vi "UTIL_SetDigitalStatus.vi"(9 "index":i32, 10 "Digital Status":T1, 11 "Cluster in":refnum<vi>) -> ()   [LabVIEW 2024]
uses:
  Control Definitions/Def_DigitalStatus.ctl
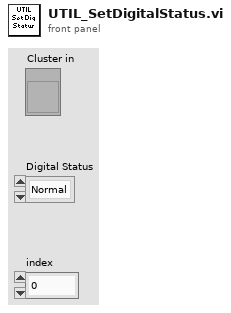
[diagram p1: front panel]
types:
  T1 = typedef "Def_DigitalStatus.ctl" = enum16{"Normal", "Good", "Bad", "Error"}
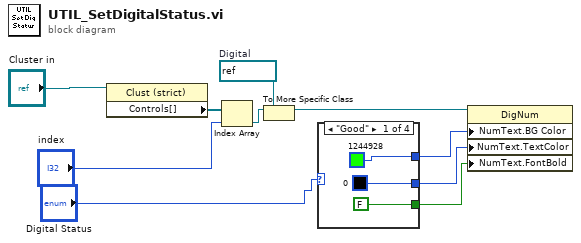
[diagram p0: block diagram]
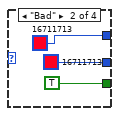
[diagram p2: hidden frame]
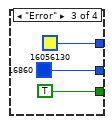
[diagram p3: hidden frame]
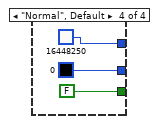
[diagram p4: hidden frame]
diagram:
  w5 = refnum<vi> refnum  # Digital
  n1 = property class="Clust (strict)"(reference="Cluster in") -> ("Controls[]"=w3:refnum<vi>[])  [unwired: 1 in, 2 out]
  n2 = Index Array(array=w3, index="index") -> (element=w4:refnum<vi>)
  n3 = To More Specific Class(target class=w5, reference=w4) -> (specific class reference=w6:refnum<vi>)  [unwired: 1 in, 1 out]
  n4 = case shown="\"Good\"" "Digital Status" {
    tunnel: [u32 0 ("Numeric Text.Colors:FG Color") u32 16711713 ("Numeric Text.Colors:FG Color") u32 16860 ("Numeric Text.Colors:FG Color") u32 0 ("Numeric Text.Colors:FG Color")] -> w9
    tunnel: [FALSE ("Numeric Text.Font:Bold") TRUE ("Numeric Text.Font:Bold") TRUE ("Numeric Text.Font:Bold") FALSE ("Numeric Text.Font:Bold")] -> w10
    tunnel: [u32 1244928 ("Numeric Text.Colors:FG Color") u32 16711713 ("Numeric Text.Colors:FG Color") u32 16056130 ("Numeric Text.Colors:FG Color") u32 16448250 ("Numeric Text.Colors:FG Color")] -> w8
    frame "Good" {
    }
    frame "Bad" {
    }
    frame "Error" {
    }
    frame "Normal", Default {
    }
  }
  n5 = property class="DigNum"(reference=w6, "NumText.BG Color"=w8, "NumText.TextColor"=w9, "NumText.FontBold"=w10) -> ()  [unwired: 1 in, 2 out]
